vi "Compressor Control.vi"() -> ()   [LabVIEW 2014]
uses:
  SRE Enum.ctl
panel:
  in  "Mode":T1
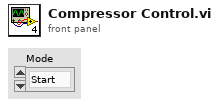
[diagram p1: front panel]
types:
  T1 = typedef "SRE Enum.ctl" = enum16{"Start", "Run", "End"}
  T2 = typedef "WPI_CompressorDevRef.ctl" = cluster{"DevStatus":errorcluster, "Pneumatics Control Module":u8}
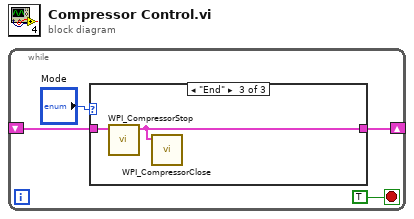
[diagram p0: block diagram]
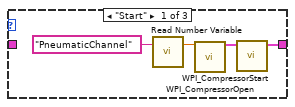
[diagram p2: hidden frame]
diagram:
  n1 = while {
    shift-right: [w3] -> _
    shift-left: _ -> [w2]
    stop <- TRUE stop-if-true
    n2 = case shown="\"End\"" "Mode" {
      tunnel: [w5 w9 w10] -> w3
      tunnel: w2 -> [_ w9 w11]
      frame "Start" {
        n3 = call "Read Number Variable.vi"("Name"="PneumaticChannel") -> ("number"=w8:dbl)  [unwired: 1 in, 1 out]
        n4 = call <vilib>:"WPI_CompressorOpen.vi"("Pneumatics Control Module (0)"=w8) -> ("CompressorDevRef"=w6:T2)  [unwired: 13 in, 1 out]
        n5 = call <vilib>:"WPI_CompressorStart.vi"("CompressorDevRef"=w6) -> ("CompressorDevRef"=w5:T2)  [unwired: 9 in, 1 out]
      }
      frame "Run", Default {
      }
      frame "End" {
        n6 = call <vilib>:"WPI_CompressorStop.vi"("CompressorDevRef"=w11) -> ("CompressorDevRef"=w10:T2)  [unwired: 9 in, 1 out]
        n7 = call <vilib>:"WPI_CompressorClose.vi"("CompressorDevRef"=w10) -> ()  [unwired: 10 in, 1 out]
      }
    }
  }
